vi "Add LVProject.vi"(8 "error in (no error)":errorcluster, 10 "Project Path":path caption="selected path", 11 "BuildServer in":refnum<class "BuildServer.lvclass">) -> (0 "error out":errorcluster, 3 "BuildServer out":refnum<class "BuildServer.lvclass">)   [LabVIEW 2017, in "BuildServer.lvlib" / "BuildServer.lvclass"]
uses:
  BuildServer.lvclass
  <vilib>/Ekim/LUT/LUT/LUT.lvclass
  <vilib>/ActorFramework/Actor/Actor.lvclass
  BuildServer Messages/Update Tree Msg/Update Tree Msg.lvclass
  Classes/Task Interface/Task/Task.lvclass
  Volumes/Data/Users/benji667/Git/BuildFarm/src/LabVIEW/vi.lib/BenjaminR/Build Farm/Actors/Framework/Actor wHelper/Actor wHelper.lvclass
  Volumes/Data/Users/benji667/Git/BuildFarm/src/LabVIEW/vi.lib/BenjaminR/Build Farm/Actors/Framework/Actor wLauncher/Actor wLauncher.lvclass
  Volumes/Data/Users/benji667/Git/BuildFarm/src/LabVIEW/vi.lib/BenjaminR/Build Farm/Actors/Framework/Actor wUI/Actor wUI.lvclass
  Applications/National Instruments/LabVIEW 2017 64-bit/vi.lib/ActorFramework/Actor/Actor.lvclass
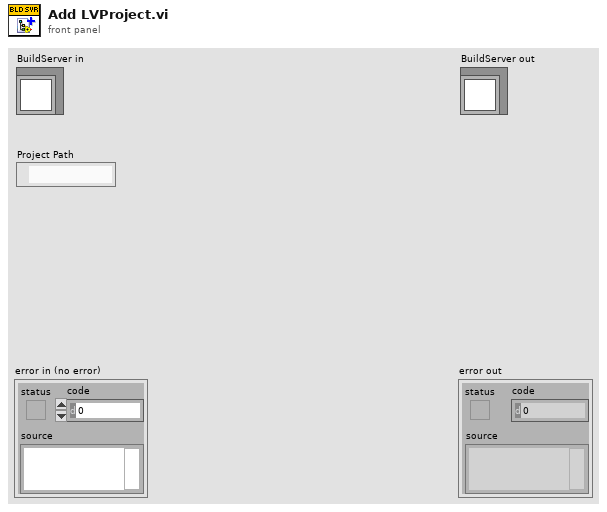
[diagram p1: front panel]
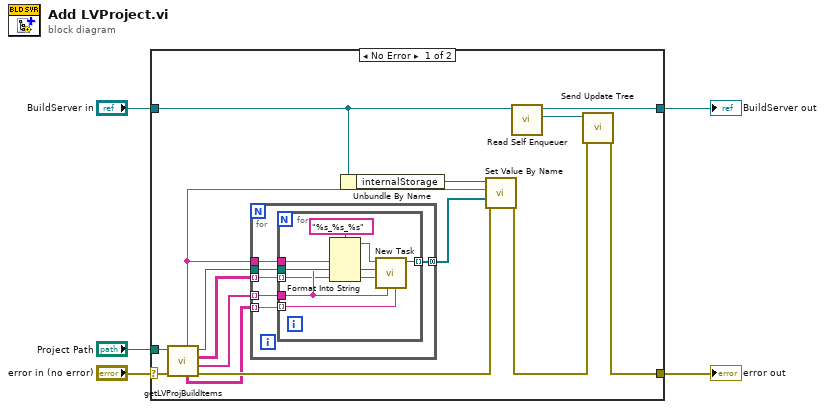
[diagram p0: block diagram]
diagram:
  n1 = case shown="No Error" "error in (no error)" {
    selector: "error in (no error)" -> [w19 w35]
    tunnel: [w10 w35] -> w4
    tunnel: [w13 w34] -> w2
    tunnel: "BuildServer in" -> [w13 w34]
    tunnel: "Project Path" -> [w6 _]
    frame No Error {
      n2 = call "getLVProjBuildItems.vi"("error in (no error)"=w19, "Project Path"=w6) -> ("error out"=w14:errorcluster, "Target Names"=w8:string[], "BuildSpec Names"=w9:string[][], "Project Path"=w16:path, "BuildSpec Type"=w7:string[][], "Project Name"=w17:string)  [unwired: 4 in]
      n3 = for {
        tunnel: w17 -> [w25]
        tunnel: w16 -> [w24]
        tunnel: w8 -> [w23] mode=indexing
        tunnel: w9 -> [w22] mode=indexing
        tunnel: [w21] -> w15 mode=concatenating
        tunnel: w7 -> [w20] mode=indexing
        n4 = for {
          tunnel: w25 -> [w30]
          tunnel: w24 -> [w33]
          tunnel: w23 -> [w29]
          tunnel: w22 -> [w28] mode=indexing
          tunnel: [w32] -> w21 mode=indexing
          tunnel: w20 -> [w31] mode=indexing
          n5 = Format Into String(format string="%s_%s_%s", w30, w29, w28) -> (resulting string=w27:string)  [unwired: 2 in, 1 out]
          n6 = call "New Task.vi"("BuildSpec Type"=w31, "Target"=w29, "BuildSpec Name"=w28, "ProjectPath"=w33, "Name"=w27) -> ("Task out"=w32:refnum<class "Task.lvclass">)  [unwired: 5 in, 1 out]
        }
      }
      n7 = Unbundle By Name(w13) -> ("internalStorage"=w18:refnum<class "LUT.lvclass">)
      n8 = call <vilib>:"Set Value By Name.vi"("error in (no error)"=w14, "Value"=w15, "Name"=w17, "LUT in"=w18) -> ("error out"=w11:errorcluster)  [unwired: 5 in, 2 out]
      n9 = call <vilib>:"Read Self Enqueuer.vi"("Actor"=w13) -> ("Self Enqueuer"=w12:refnum<class "Message Enqueuer.lvclass">)  [unwired: 10 in]
      n10 = call "Send Update Tree.vi"("error in (no error)"=w11, "Message Enqueuer in"=w12) -> ("error out"=w10:errorcluster)  [unwired: 8 in, 1 out]
    }
    frame Error {
    }
  }
  "error out" <- w4
  "BuildServer out" <- w2
